vi "destroyer Events.vi"(8 "error in (no error)":errorcluster, 11 "Measurement Señal Actualizable in":refnum<class "Measurement Señal Actualizable.lvclass">) -> (0 "error out":errorcluster, 3 "Measurement Señal Actualizable out":refnum<class "Measurement Señal Actualizable.lvclass">)   [LabVIEW 2020, in "Measurement Señal Actualizable.lvlib" / "Measurement Señal Actualizable.lvclass"]
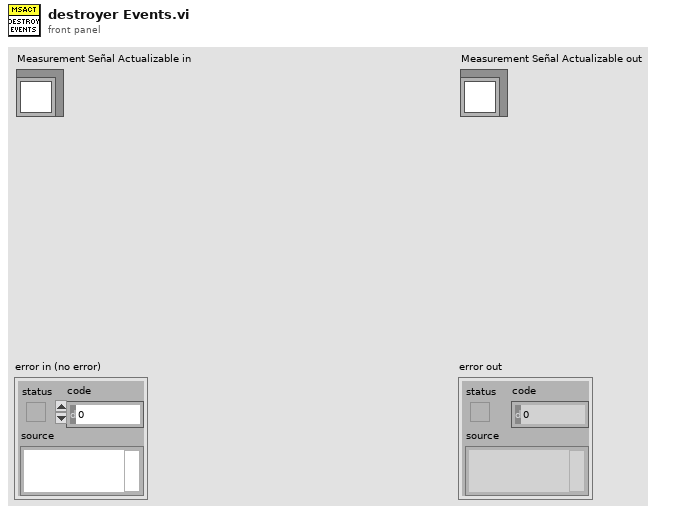
[diagram p1: front panel]
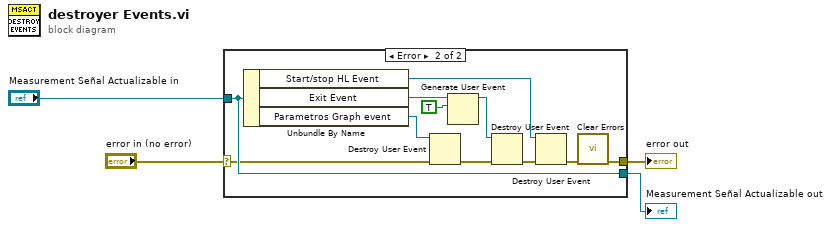
[diagram p0: block diagram]
diagram:
  n1 = case shown="Error" "error in (no error)" {
    selector: "error in (no error)" -> [w5 w11]
    tunnel: [w5 w7] -> w3
    tunnel: [w6 w17] -> w1
    tunnel: "Measurement Señal Actualizable in" -> [w6 w17]
    frame No Error {
    }
    frame Error {
      n2 = Unbundle By Name(w17) -> ("Start/stop HL Event"=w16:refnum<user-event>, "Exit Event"=w15:refnum<user-event>, "Parametros Graph event"=w12:refnum<user-event>)
      n3 = Destroy User Event(user event=w12, error in=w11) -> (error out=w10:errorcluster)
      n4 = Generate User Event(user event=w15, event data cluster=TRUE ("event data")) -> (user event out=w13:refnum<user-event>)  [unwired: 2 in, 1 out]
      n5 = Destroy User Event(user event=w13, error in=w10) -> (error out=w9:errorcluster)
      n6 = Destroy User Event(user event=w16, error in=w9) -> (error out=w8:errorcluster)
      n7 = call <vilib>:"Clear Errors.vi"("error in (no error)"=w8) -> ("error out"=w7:errorcluster)  [unwired: 5 in, 1 out]
    }
  }
  "error out" <- w3
  "Measurement Señal Actualizable out" <- w1
